vi "VI Interference Konfig.vi"() -> ()   [LabVIEW 2020, in "EPA 1065.lvlib" / "Interference verificaton 1065-375.lvlib"]
uses:
  Interference verificaton 1065-375.lvlib
  Visualisierungs Elemente/Zahlen-Ausgabefeld.ctl
  ResultTable.ctl
  TestKonfig.ctl
  Modus.ctl
  TestSetting.ctl
  Seiten/System Einstellungen V2/Analysatoren.ctl
  Visualisierungs Elemente/String - Ausgabefeld.ctl
  Aktion Test.ctl
  Aktion FGV Interference.ctl
  Linearisierung V2/AktivButton.ctl
  Sprachverwaltung/FGV Aktion Tabelle zerlegen.ctl
  Seiten/FT-IR/FGV FT-IR Gasliste Aktionen.ctl
  Aktion Index uebersetzten.ctl
  Allgemeine VIs/Aktion Test Status.ctl
  Allgemeine VIs/Aktion Wertaenderung Gasliste.ctl
  Messdaten/Aktionen FGV Messdaten.ctl
  Funktionstasten/Zustaende.ctl
  Funktionstasten/Funktionstasten-Aktion.ctl
  <vilib>/Utility/miscctls.llb/LVRowAndColumnTypeDef.ctl
  Seiten/FT-IR/FGV FT-IR Parameter.vi
  Messdaten/Messdaten.lvlib
  Seiten/Grafik/Grafik.lvlib
  Allgemein/allgemeine Sub-VIs.lvlib
  Seiten/FT-IR/FT-IR.lvlib
  Sprachverwaltung/Sprachverwaltung.lvlib
  Funktionstasten/Funktionstasten.lvlib
  Linearisierung V2/Protokoll/Protokoll.lvlib
  Seiten/FT-IR/Span/Spanfaktor.lvlib
  Linearisierung V2/Linearisierung v2.lvlib
  EPA 1065.lvlib
  Seiten/System Einstellungen V2/System Einstellungen V2.lvlib
panel:
  in  "Systemeinstellung":bool caption="Gasliste geändert"
  out "max. Flow Weighted Mean:":T1 caption="ppm"
  out "Konzentration FlowWeightedMean":sgl=120.0 caption="Konzentration:" min=0 format="%#.2f"
  in  "Gasliste vergleichen":bool
  in  "Registerkarte":T2(tab)
  in  "Speichern 2":bool caption="Speichern"
  in  "TestSetting":T3={"Bearbeiter:"="", "Pfad:"=path "D:/IAG_Data/Log", "Textname:"="", "Analysator"=""}
  in  "TestKonfig":T5={"Komponente:"=0, "Modus"=0, "CG Aufschaltzeit:"=120.0, "Interferent 1:"=0, "Interferent 2:"=0, "Interferent 3:"=0, "Gasflaschen Nr.:"="", "Gasflaschen Nr.: 2"="", "Gasflaschen Nr.: 3"="", "Inter 1 aktiv"=FALSE, "Inter 2 aktiv"=FALSE, "Inter 3 aktiv"=FALSE, "Accuracy"="", "Accuracy 2"="", "Accuracy 3"="", "Konzentration 1:"=120.0, "Konzentration 2:"=120.0, "Konzentration 3:"=120.0} {"Komponente:" items=["N2O (300) LP 191C (1of2)", "N2O (1000) LP 191C (2of2)", "N2O autorange (1000)"]; "Konzentration 3:" min=0.0; "Interferent 3:" items=["CO% (1) LP 191C (2of3)", "CO% (10) LP 191C (3of3)", "HNCO (400) 191C", "CO (700) LP 191C (1of3)", "CO autorange (100000)"]; "Konzentration 2:" min=0.0; "Interferent 2:" items=["H2O% (30) LP 191C", "H2Oppm (300000)"]; "Konzentration 1:" min=0.0; "Interferent 1:" items=["CO2 low% (4) LP 191C (2of2)", "CO2% (20) LP 191C (1of2)", "CO2% autorange (20)"]; "Modus" items=["Messen", "CG zu Entnahmestelle"]; "CG Aufschaltzeit:" min=60.0}
  in  "Speichern":bool
  in  "Graph löschen":bool caption="Test Start"
  out "Interferent 3:":T1
  out "Interferent 3: 2":T7 caption="ppm" format="%#.2f"
  out "Interferent 2:":T1
  out "Interferent 2: 2":T7 caption="%" format="%#.2f"
  out "Interferent 1:":T1
  out "Interferent 1: 2":T7 caption="%" format="%#.2f"
  in  "Abbrechen":bool caption="Test Start"
  out "Testdauer":T7
  out "Stabilisierungszeit":T7
  out "Graph":waveform(dbl)[](graph)
  out "Status":string
  in  "Test Start":bool
  out "Komponente 1S:":T1 caption="Komponente:"
  out "Komponente 1:":T7 caption="ppm" format="%#.2f"
  in  "Save to file":bool caption="PDF erstellen"
  out "[ppm]":sgl=1.0 caption="Grenze:" min=0 format="%#.6g"
  out "[ppm]":sgl=120.0 caption="Querempfindlichkeit:" min=0 format="%#.6g"
  out "Konzentration Komponente":sgl=120.0 caption="Konzentration:" min=0 format="%#.2f"
  out "Komponente:":T1 caption="ppm"
  out "LIN Ausgabetabelle":T8
  in  "Daten löschen":bool caption="Test Start"
  in  "Print to PDF":bool caption="PDF erstellen"
  out "Tabelle 3":string[][](table)
  # "N2O Querempfindlichkeitsnachweis 1065.375"
  # "Interference Test"
  # "Interference Verification"
  # "max. Flussgewichteter Mittelwert"
  # "Einstellungen"
  # "General Information"
  # "Report Settings"
  # "Test Einstellungen"
  # "Komponente:"
  # "Interferenten"
  # "sec."
  # "Test"
  # "Ergebnis"
  # "Analyse"
  # "Komponente:"
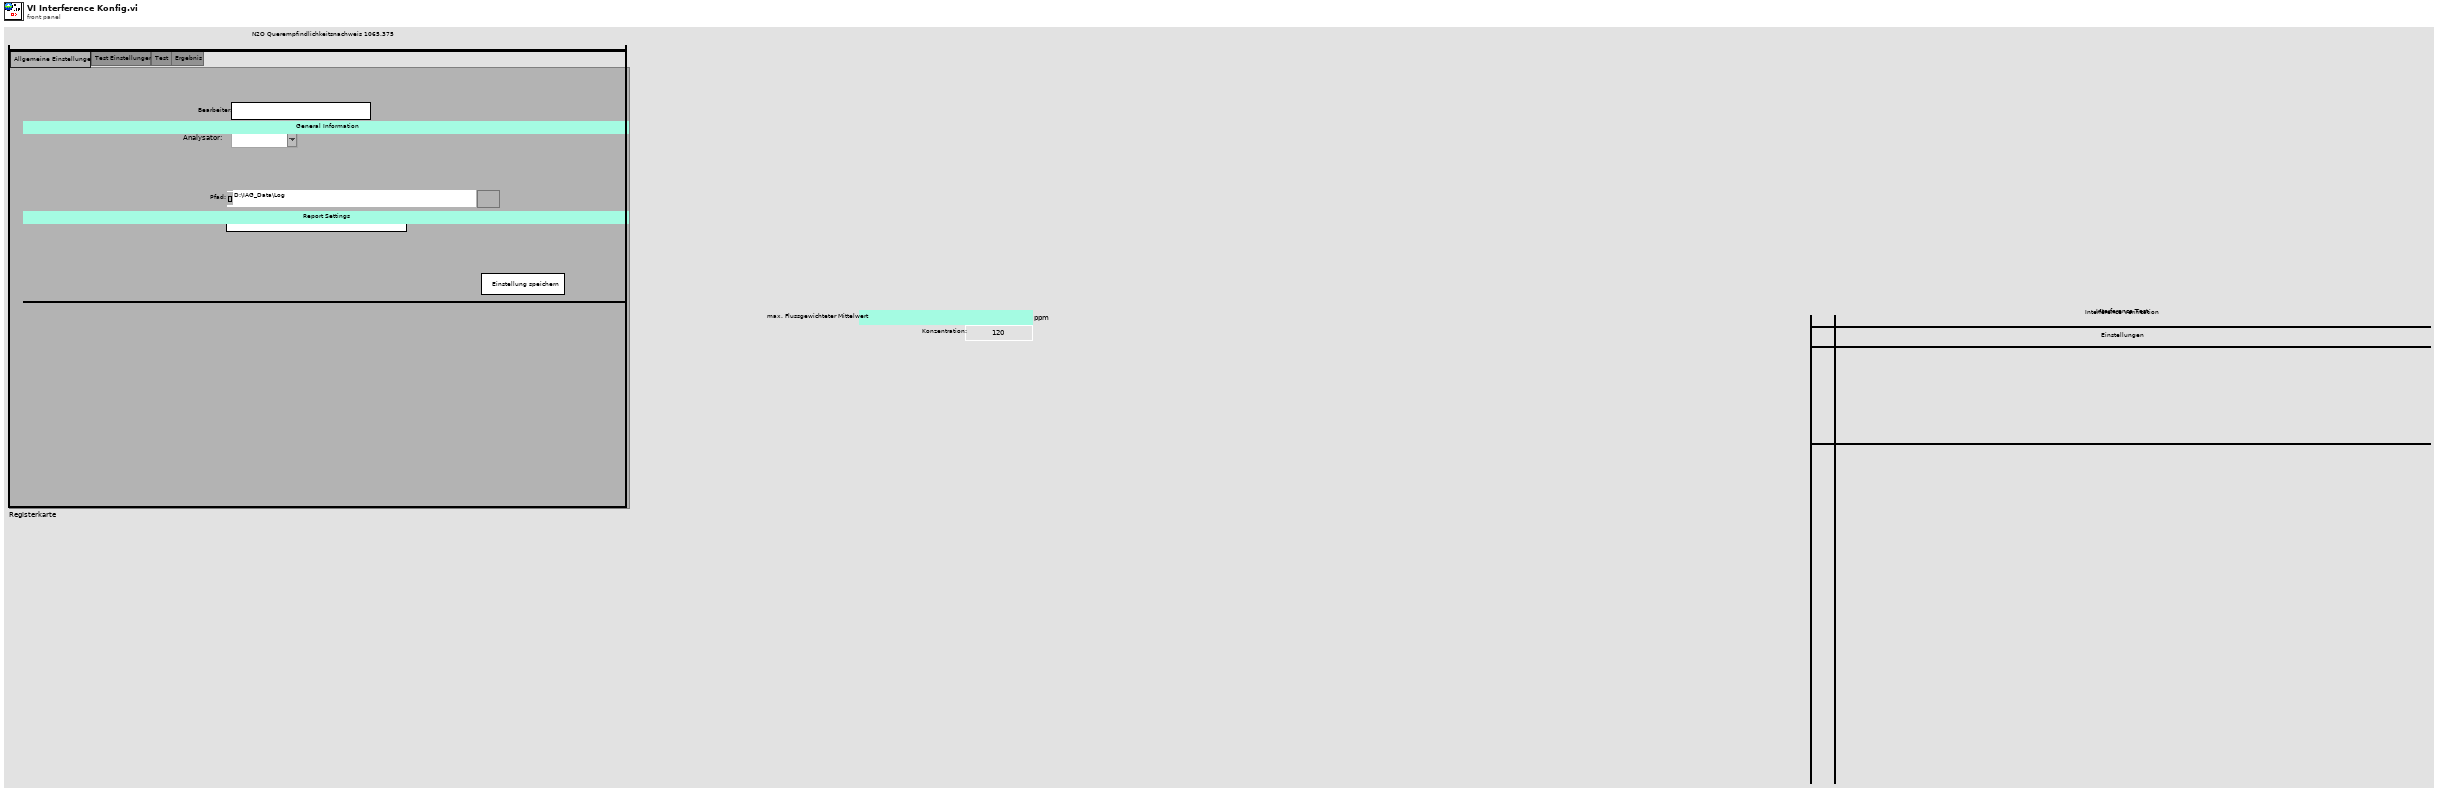
[diagram p1: front panel]
types:
  T1 = typedef "String - Ausgabefeld.ctl" = string
  T2 = enum32{"General Settings", "Test Settings", "Test", "Result"}
  T3 = typedef "EPA 1065.lvlib/Interference verificaton 1065-375.lvlib/TestSetting.ctl" = cluster{"Bearbeiter:":string, "Pfad:":path, "Textname:":string, "Analysator":T4}
  T4 = typedef "System Einstellungen V2.lvlib/Analysatoren.ctl" = string
  T5 = typedef "EPA 1065.lvlib/Interference verificaton 1065-375.lvlib/TestKonfig.ctl" = cluster{"Komponente:":u16, "Modus":T6, "CG Aufschaltzeit:":dbl, "Interferent 1:":u16, "Interferent 2:":u16, "Interferent 3:":u16, "Gasflaschen Nr.:":string, "Gasflaschen Nr.: 2":string, "Gasflaschen Nr.: 3":string, "Inter 1 aktiv":bool, "Inter 2 aktiv":bool, "Inter 3 aktiv":bool, "Accuracy":string, "Accuracy 2":string, "Accuracy 3":string, "Konzentration 1:":dbl, "Konzentration 2:":dbl, "Konzentration 3:":dbl}
  T6 = typedef "EPA 1065.lvlib/Interference verificaton 1065-375.lvlib/Modus.ctl" = u16
  T7 = typedef "Zahlen-Ausgabefeld.ctl" = sgl
  T8 = typedef "EPA 1065.lvlib/Interference verificaton 1065-375.lvlib/ResultTable.ctl" = string[][]
  T9 = typedef "EPA 1065.lvlib/Interference verificaton 1065-375.lvlib/Aktion Test.ctl" = enum16{"Lesen", "ini", "ini - Konz", "Konzentration erreicht", "ini-warten", "ini-Warten-Stabil", "Warten-Stabil", "ini-warten-aufzeichnen", "Warten-Aufzeichnen", "aufzeichnen", "ini-wet", "ini - konz - wet", "Konzentration erreicht - wet", "ini - warten - wet", "warten - wet", "warten - aufzeichnen - wet", "Auswerten", "aufzeichnen - wet"}
  T10 = typedef "Sprachverwaltung.lvlib/FGV Aktion Tabelle zerlegen.ctl" = enum16{"laden", "vereinzeln", "speichern"}
  T11 = typedef "Linearisierung v2.lvlib/AktivButton.ctl" = bool
  T12 = typedef "EPA 1065.lvlib/Interference verificaton 1065-375.lvlib/Aktion FGV Interference.ctl" = enum16{"Lesen", "TestKonfig", "TestSetting", "Einheiten", "Ergebnis", "Laden", "Tabelle", "Speichern", "löschen"}
  T13 = enum8{"Enabled", "Disabled", "Disabled and Grayed Out"}
  T14 = typedef "EPA 1065.lvlib/Interference verificaton 1065-375.lvlib/Aktion Index uebersetzten.ctl" = enum16{"lesen", "schreiben", "auswerten"}
  T15 = typedef "FT-IR.lvlib/FGV FT-IR Gasliste Aktionen.ctl" = enum16{"lesen", "Gasliste FT-IR", "Gasliste ausgelesen", "laden", "speichern", "löschen"}
  T16 = typedef "EPA 1065.lvlib/Interference verificaton 1065-375.lvlib/Komponenten.ctl" = cluster{"Komponente":T1, "Komponente Index":i32, "Komponente 2":T1, "Komponente Index 2":i32, "Komponente 3":T1, "Komponente Index 3":i32, "Interferent 1":T1, "Interferent Index":i32, "Interferent 2":T1, "Interferent 2 Index":i32, "Interferent 3":T1, "Interferent 3 Index":i32, "Interferent 4":T1, "Interferent 4 Index":i32}
  T17 = typedef "EPA 1065.lvlib/Aktion Wertaenderung Gasliste.ctl" = enum16{"Init", "lesen", "Gasliste geändert", "ARN inaktiv", "LEAK inaktiv", "Interference 366 inaktiv", "T90 inaktiv", "Interference 375 inaktiv", "Chiller inaktiv", "FID O2 inaktiv", "FID Opti inaktiv", "Drift inaktiv", "Pre Test inaktiv", "LinV2 inaktiv", "HovaCAL Interference inaktiv"}
  T18 = typedef "EPA 1065.lvlib/Aktion Test Status.ctl" = enum16{"init", "lesen", "prüfen", "Interference 366", "Interference 375", "Chiller läuft", "Drift läuft", "Pre Test läuft", "FID Optimization läuft", "FID Interference läuft", "HovaCAL Interference", "LinV2"}
  T19 = typedef "Messdaten.lvlib/Aktionen FGV Messdaten.ctl" = enum16{"lesen", "schreiben", "löschen", "Mittelwerte", "Komponente"}
  T20 = typedef "Funktionstasten.lvlib/Funktionstasten-Aktion.ctl" = enum16{"Initialisieren", "Zustand setzen", "Taste gedrückt", "Fehler speichern", "Lesen", "Manuell", "Remote", "Bitparallel", "Samplepoint", "Zeit Prüfen", "reset Umschalten"}
  T21 = typedef "Funktionstasten.lvlib/Zustaende.ctl" = enum16{"Standby", "Pause", "Eco", "Messen", "Kalibrieren", "Spülen Filter", "Spülen Leitung", "Umgebungsluft", "0-Gas", "Cal-Gas", "CG zu PNS", "-------------", "Init 1", "Init 2", "Init 3", "Init 4", "Messen vorbereiten", "Messen durchführen", "Exit"}
  T22 = enum16{"open", "replace", "create", "open or create", "replace or create", "replace or create with confirmation"}
  T23 = typedef "LVRowAndColumnTypeDef.ctl" = cluster{"Row":i32, "Column":i32}
  T24 = typedef "EPA 1065.lvlib/Aktive Tests Cluster.ctl" = cluster{"ANR läuft":bool, "T90 läuft":bool, "Leak läuft":bool, "Interference 366 läuft":bool, "Interference 375 läuft":bool, "Chiller läuft":bool, "FID Interference läuft":bool, "FID optimization läuft":bool, "Drift läuft":bool, "Pre-test läuft":bool, "HovaCAL Interference läuft":bool, "LinV2 läuft":bool}
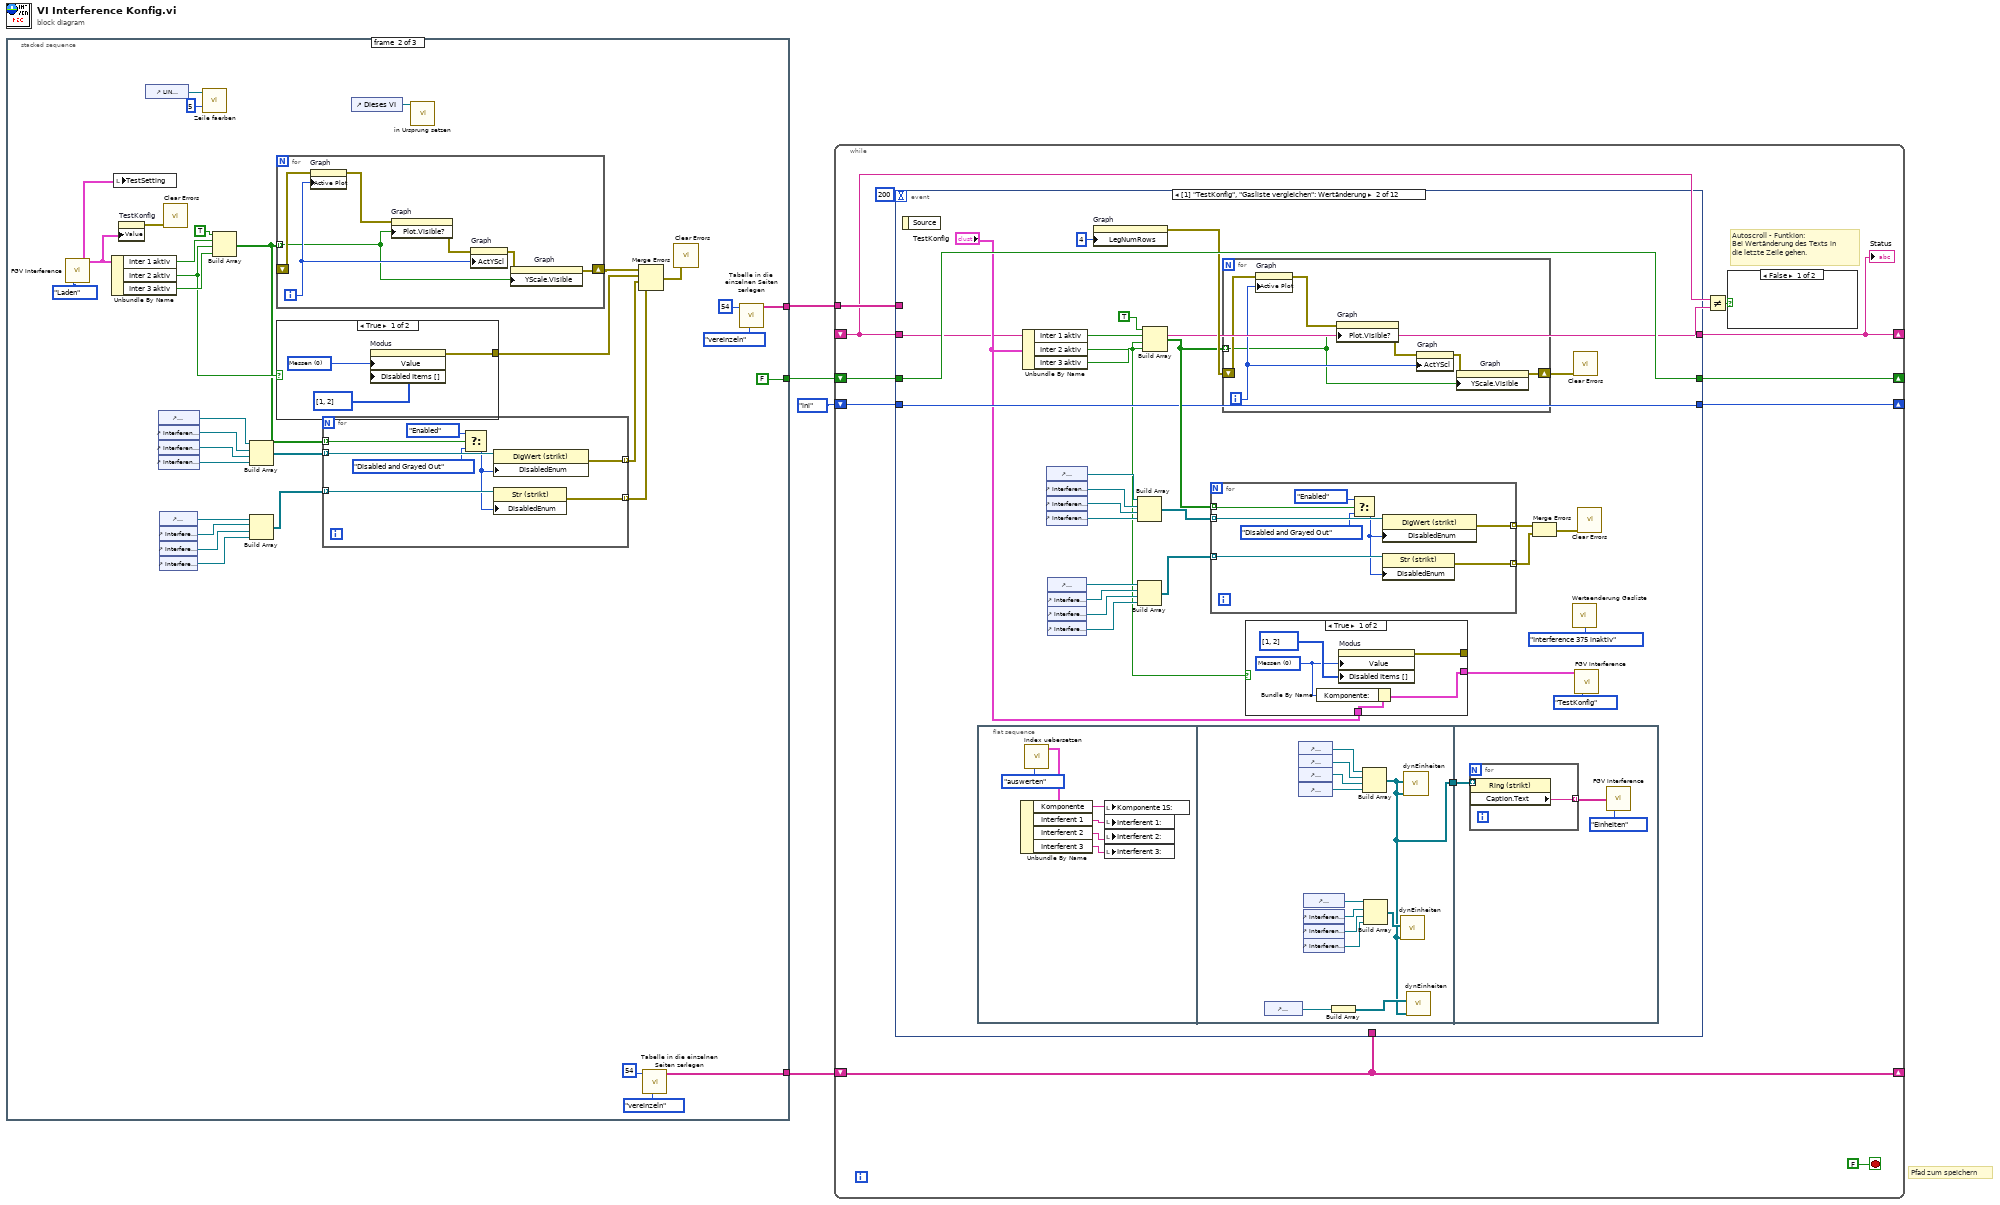
[diagram p0: block diagram]
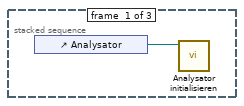
[diagram p2: hidden frame]
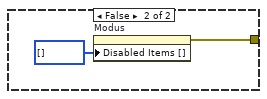
[diagram p3: hidden frame]
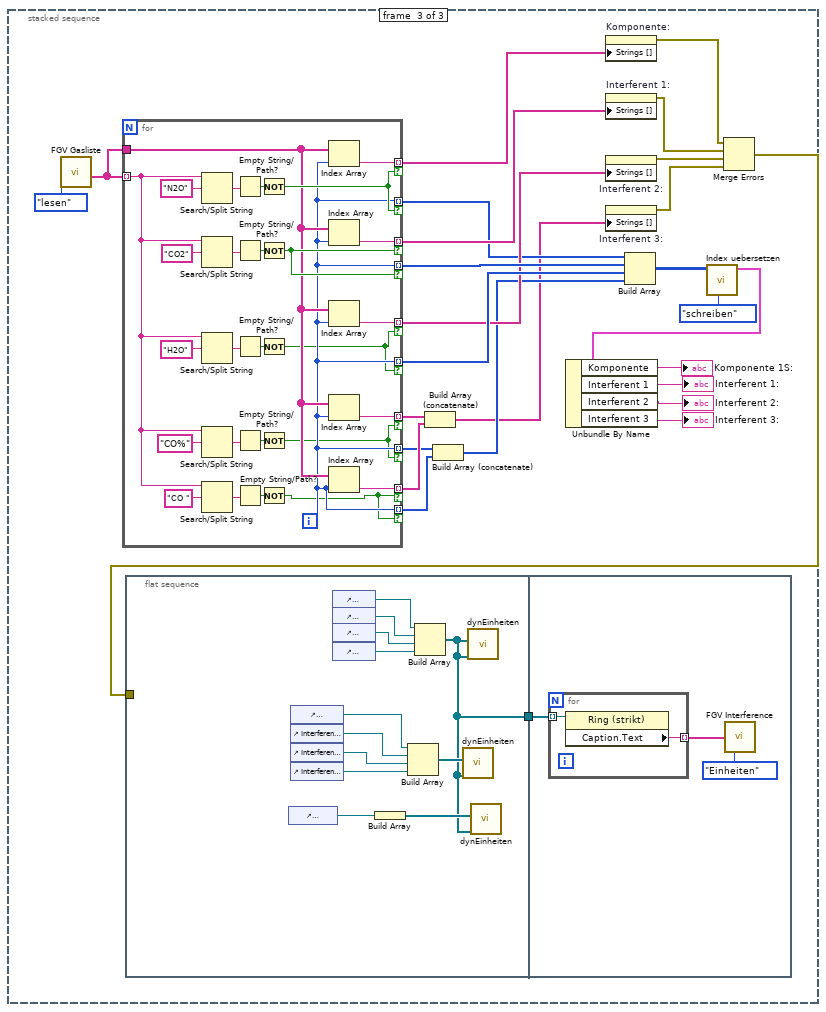
[diagram p4: hidden frame]
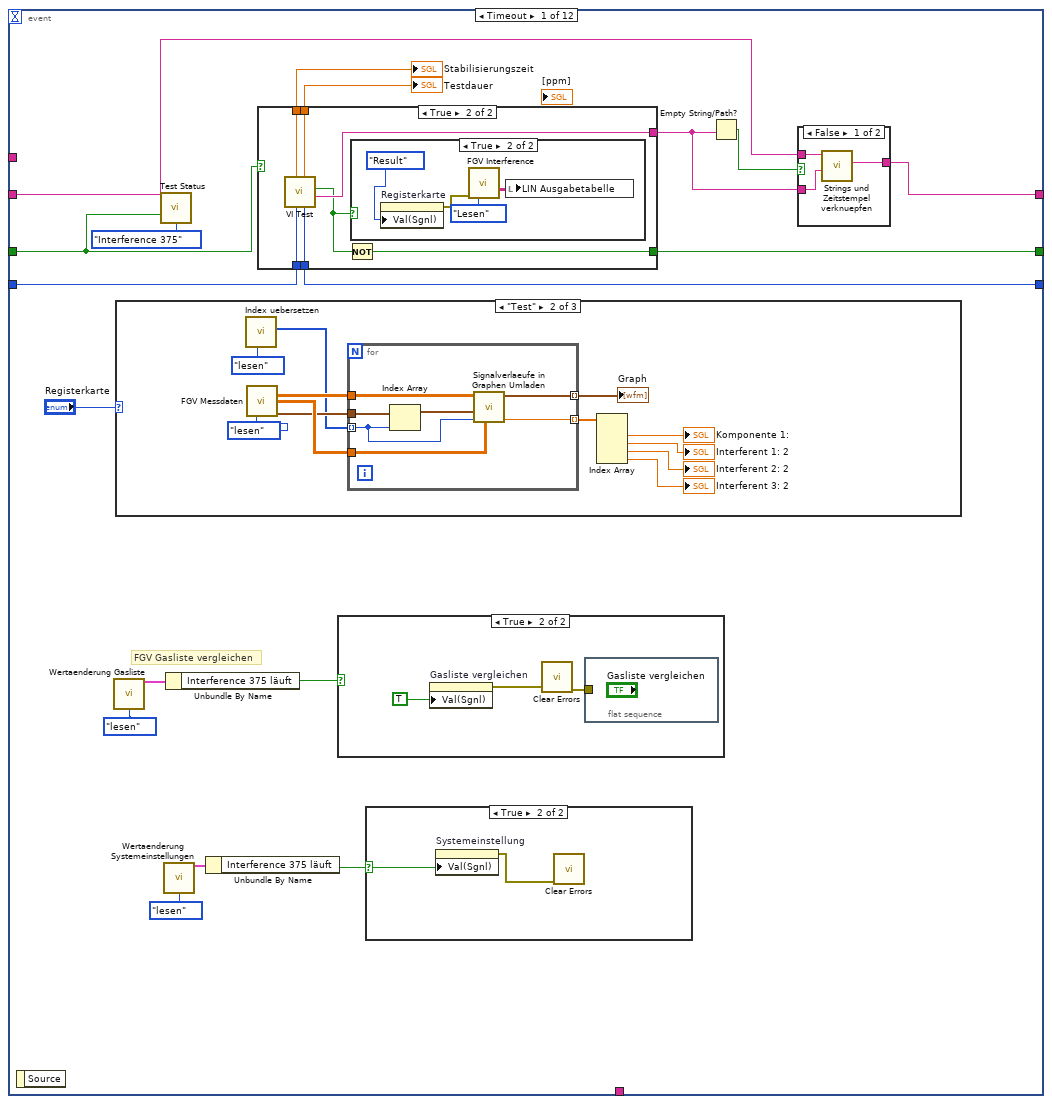
[diagram p5: hidden frame]
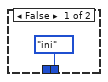
[diagram p10: hidden frame]
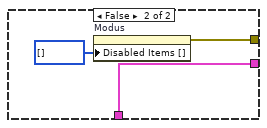
[diagram p13: hidden frame]
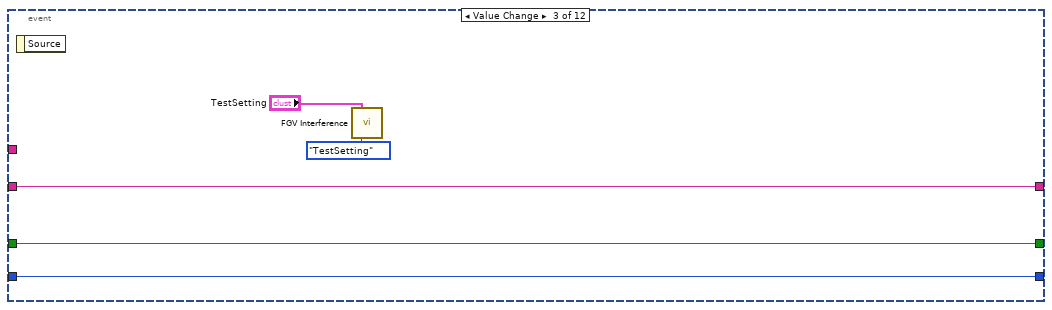
[diagram p14: hidden frame]
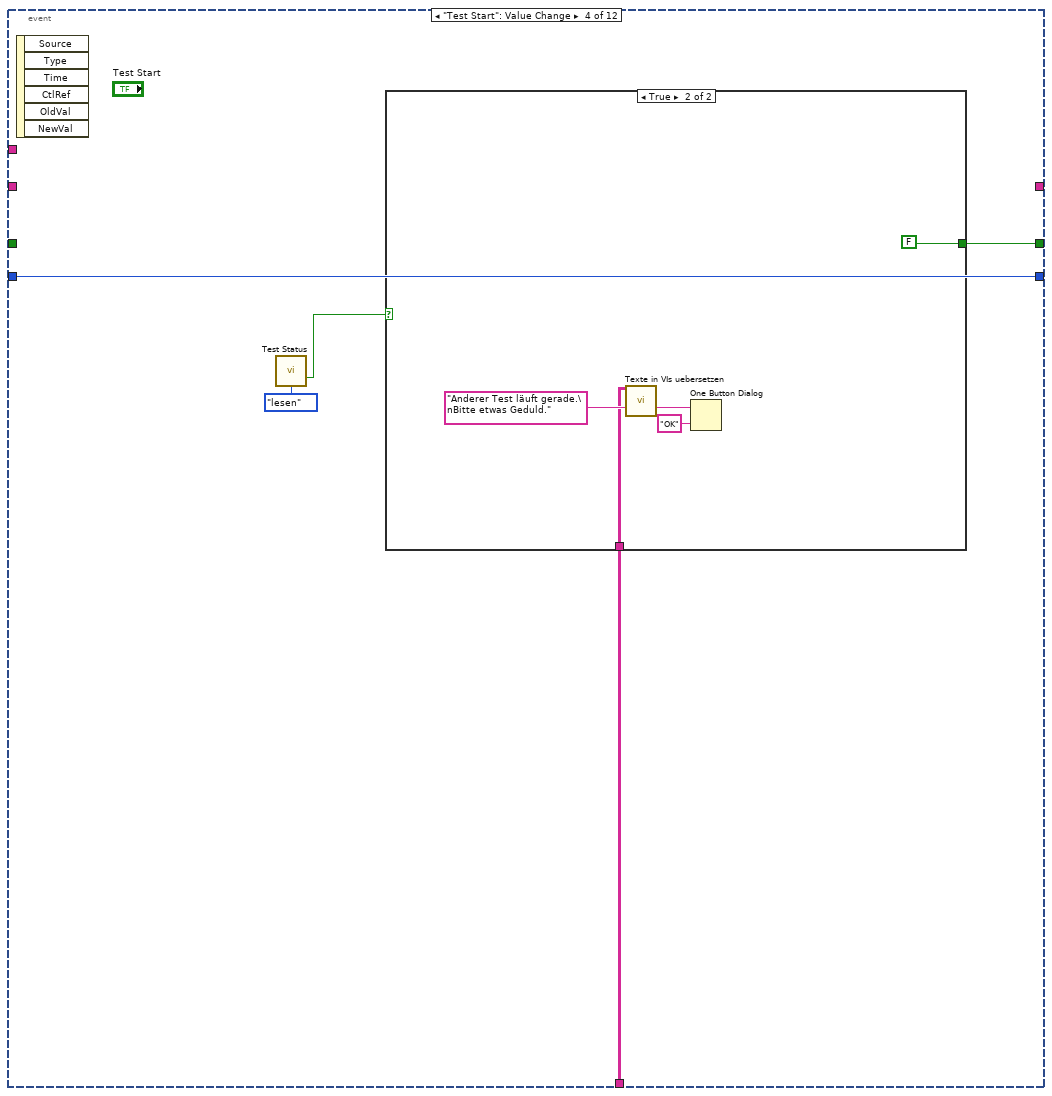
[diagram p15: hidden frame]
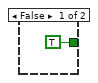
[diagram p16: hidden frame]
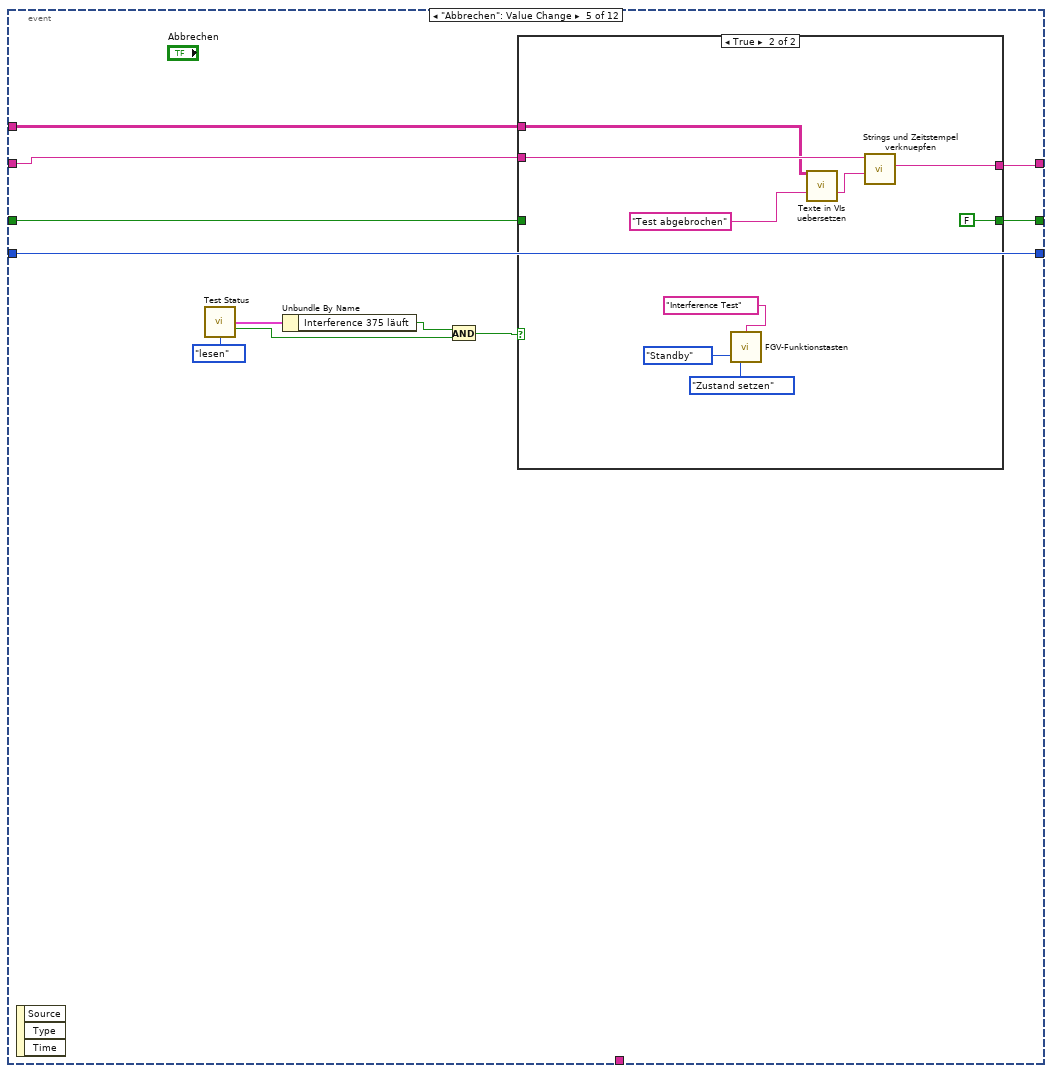
[diagram p17: hidden frame]
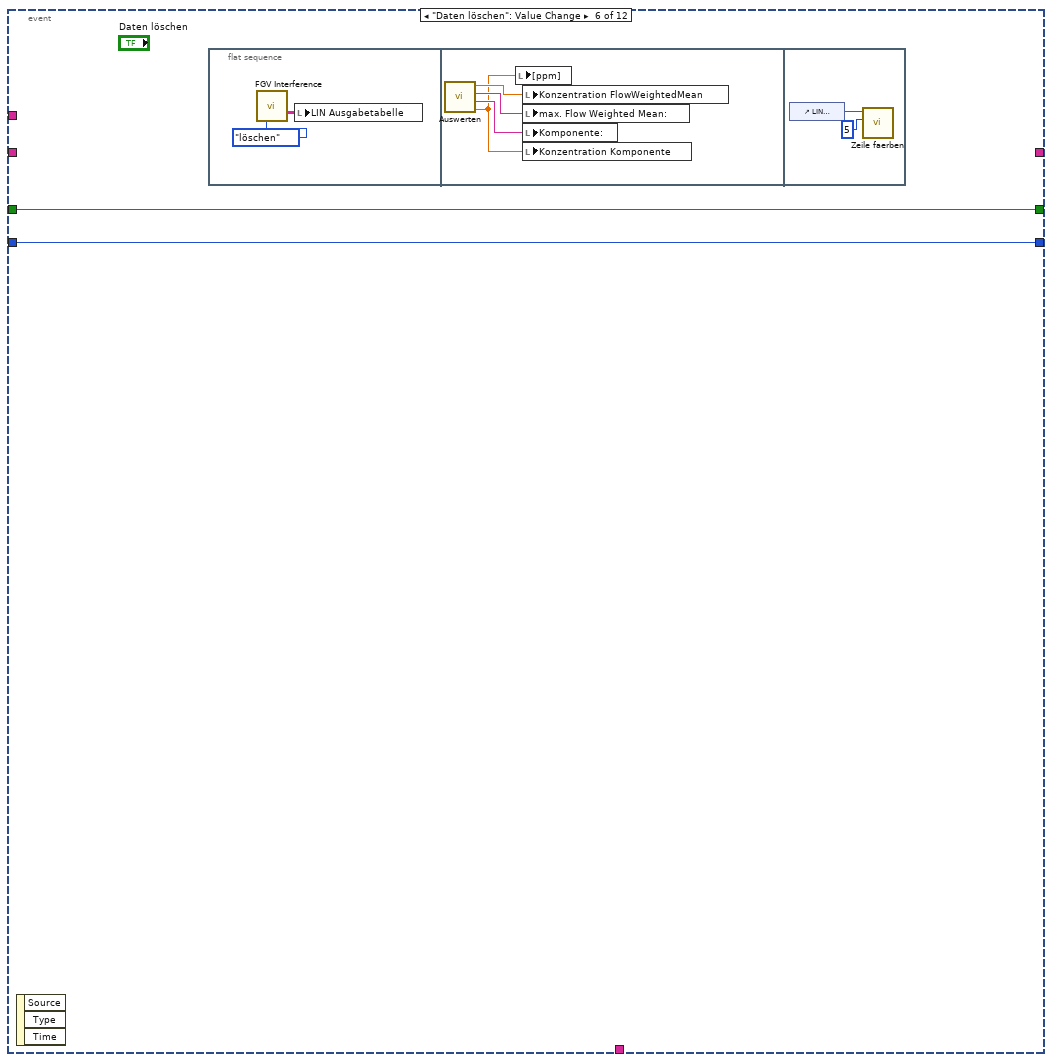
[diagram p19: hidden frame]
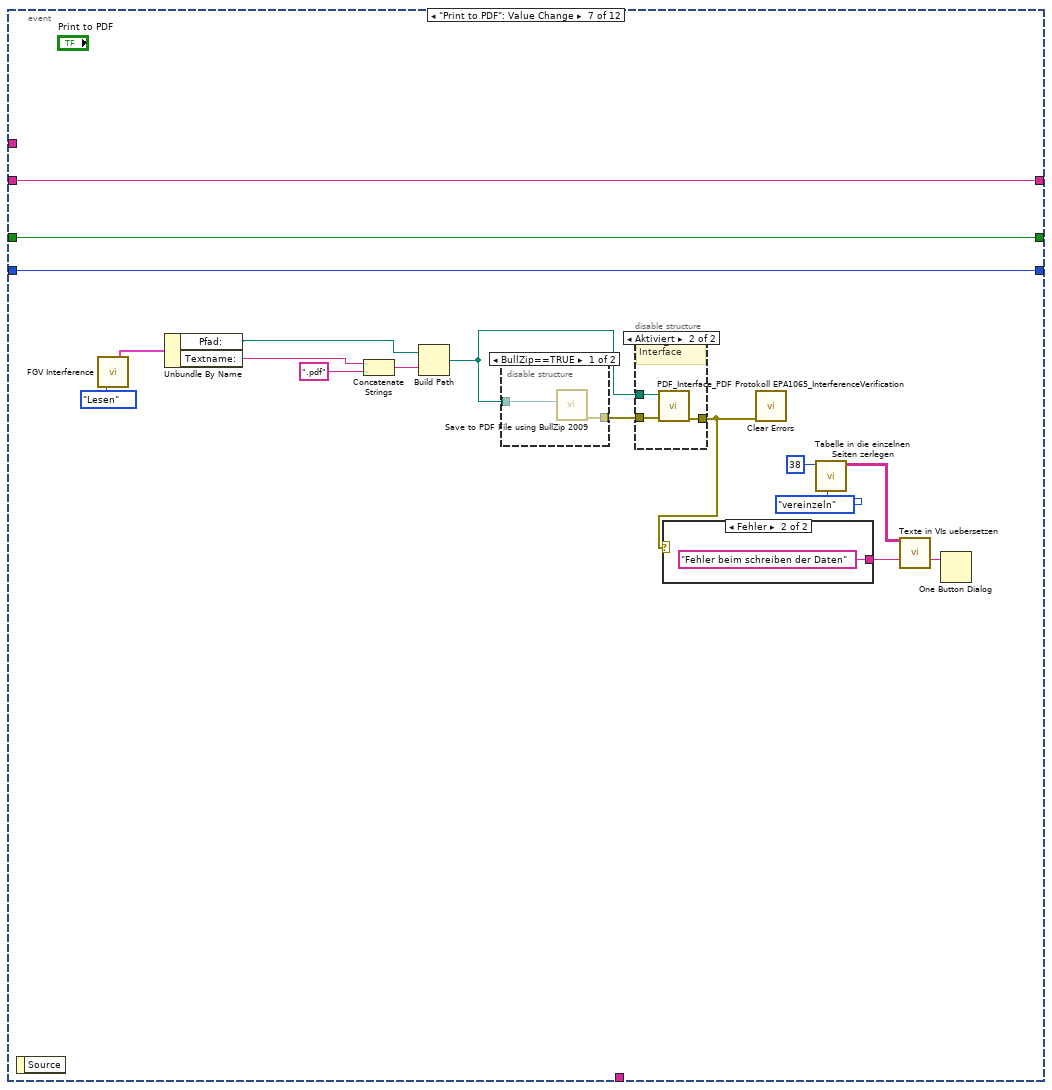
[diagram p20: hidden frame]
diagram:
  # "Pfad zum speichern"
  n1 = stacked-sequence {
    tunnel: [_ w37 _] -> w4
    tunnel: [_ FALSE _] -> w3
    tunnel: [_ w19 _] -> w1
    frame #0 {
      n2 = control-ref of="Analysator"() -> (w5:refnum<vi>)
      n3 = call "Analysator initialisieren.vi"("Referenz Analysator"=w5) -> ()  [unwired: 9 in, 2 out]
    }
    frame #1 {
      n4 = call "FGV Interference.vi"("Aktion FGV Interference"=Aktion_FGV_Interference."Laden") -> ("TestSetting"=w30:T3, "TestKonfig 2"=w34:T5)  [unwired: 9 in, 4 out]
      n5 = Unbundle By Name(w34) -> ("Inter 1 aktiv"=w29:bool, "Inter 2 aktiv"=w25:bool, "Inter 3 aktiv"=w28:bool)
      n6 = local write "TestSetting"(w30) -> ()
      n7 = property on="TestKonfig" class="Cluster (strikt)"("Value"=w34) -> (error out=w33:errorcluster)  [unwired: 2 in, 1 out]
      n8 = control-ref of="LIN Ausgabetabelle"() -> (w31:refnum<vi>)
      n9 = control-ref of="Komponente 1:"() -> (w12:refnum<vi>)
      n10 = control-ref of="Interferent 1: 2"() -> (w11:refnum<vi>)
      n11 = control-ref of="Interferent 2: 2"() -> (w10:refnum<vi>)
      n12 = control-ref of="Interferent 3: 2"() -> (w9:refnum<vi>)
      n13 = control-ref of="Komponente 1S:"() -> (w13:refnum<vi>)
      n14 = control-ref of="Interferent 1:"() -> (w14:refnum<vi>)
      n15 = control-ref of="Interferent 2:"() -> (w15:refnum<vi>)
      n16 = control-ref of="Interferent 3:"() -> (w16:refnum<vi>)
      n17 = call <vilib>:"Clear Errors.vi"("error in (no error)"=w33) -> ()  [unwired: 5 in, 2 out]
      n18 = call "Zeile faerben.vi"("Anzahl"=5, "Table (Eingang)"=w31) -> ()  [unwired: 9 in, 1 out]
      n19 = Build Array(T11 TRUE ("Element"), w29, w25, w28) -> (w8:T11[])
      n20 = Build Array(w12, w11, w10, w9) -> (w17:refnum<vi>[])
      n21 = Build Array(w13, w14, w15, w16) -> (w18:refnum<vi>[])
      n22 = for {
        shift-right: [w56] -> w24
        shift-left: _ -> [w55]
        tunnel: w8 -> [w53] mode=indexing
        i -> [w54]
        n23 = property on="Graph" class="SVDiagr (strikt)"(error in=w55, "Active Plot"=w54) -> (error out=w57:errorcluster)  [unwired: 1 in, 1 out]
        n24 = property on="Graph" class="SVDiagr (strikt)"(error in=w57, "Plot.Visible?"=w53) -> (error out=w58:errorcluster)  [unwired: 1 in, 1 out]
        n25 = property on="Graph" class="SVDiagr (strikt)"(error in=w58, "ActYScl"=w54) -> (error out=w59:errorcluster)  [unwired: 1 in, 1 out]
        n26 = property on="Graph" class="SVDiagr (strikt)"(error in=w59, "YScale.Visible"=w53) -> (error out=w56:errorcluster)  [unwired: 1 in, 1 out]
      }
      n27 = case shown="True" w25 {
        tunnel: [w48 w51] -> w22
        frame True {
          w50 = T6 0 items=["Messen", "CG zu PNS", "CG zu Entnahmestelle"] ("Wert")
          n28 = property on="Modus" class="Ring (strikt)"("Value"=w50, "Disabled Items []"=i32[] [1, 2] ("Deaktivierte Objekte []")) -> (error out=w48:errorcluster)  [unwired: 2 in, 1 out]
        }
        frame False {
          n29 = property on="Modus" class="Ring (strikt)"("Disabled Items []"=i32[] [] ("Deaktivierte Objekte []")) -> (error out=w51:errorcluster)  [unwired: 2 in, 1 out]
        }
      }
      n30 = for {
        tunnel: w8 -> [w40] mode=indexing
        tunnel: w17 -> [w47] mode=indexing
        tunnel: w18 -> [w46] mode=indexing
        tunnel: [w45] -> w7 mode=indexing
        tunnel: [w44] -> w6 mode=indexing
        n31 = Select(t=T13."Enabled" ("Deaktiviert"), s=w40, f=T13."Disabled and Grayed Out" ("Deaktiviert")) -> (s? t:f=w41:T13)
        n32 = property class="DigWert (strikt)"(reference=w47, "DisabledEnum"=w41) -> (error out=w45:errorcluster)  [unwired: 1 in, 1 out]
        n33 = property class="Str (strikt)"(reference=w46, "DisabledEnum"=w41) -> (error out=w44:errorcluster)  [unwired: 1 in, 1 out]
      }
      n34 = control-ref of="Dieses VI"() -> (w39:refnum<vi>)
      n35 = call "in Ursprung setzen.vi"("VI Referenz"=w39) -> ()  [unwired: 10 in, 1 out]
      n36 = Merge Errors(w24, w22, w7, w6) -> (w23:errorcluster)
      n37 = call "Tabelle in die einzelnen Seiten zerlegen.vi"("Aktion"=FGV_Aktion_Tabelle_zerlegen."vereinzeln", "Index (Seite)"=54) -> ("Sprachliste"=w19:string[][])  [unwired: 7 in, 2 out]
      n38 = call <vilib>:"Clear Errors.vi"("error in (no error)"=w23) -> ()  [unwired: 5 in, 2 out]
      n39 = call "Tabelle in die einzelnen Seiten zerlegen.vi"("Aktion"=FGV_Aktion_Tabelle_zerlegen."vereinzeln", "Index (Seite)"=54) -> ("Sprachliste"=w37:string[][])  [unwired: 7 in, 2 out]
    }
    frame #2 {
      n40 = call "FGV Gasliste.vi"("Aktionen"=FGV_FT-IR_Gasliste_Aktionen."lesen") -> ("Aktuelle Gasliste gesamt"=w83:T1[])  [unwired: 8 in, 2 out]
      n41 = for {
        tunnel: w83 -> [w110] mode=indexing
        tunnel: w83 -> [w109]
        tunnel: [w128] -> w69 mode=indexing if=w127
        tunnel: [w107] -> w66 mode=indexing if=w127
        tunnel: [w125] -> w68 mode=indexing if=w126
        tunnel: [w107] -> w73 mode=indexing if=w126
        tunnel: [w118] -> w67 mode=indexing if=w105
        tunnel: [w107] -> w84 mode=indexing if=w105
        tunnel: [w117] -> w65 mode=indexing if=w106
        tunnel: [w107] -> w63 mode=indexing if=w106
        tunnel: [w108] -> w64 mode=indexing if=w104
        tunnel: [w107] -> w62 mode=indexing if=w104
        i -> [w107]
        n42 = Search/Split String(string=w110, search string/char (-)="N2O" ("Such-String/-Zeichen (-)")) -> (match + rest of string=w130:T1)  [unwired: 1 in, 2 out]
        n43 = Search/Split String(string=w110, search string/char (-)="CO2" ("Such-String/-Zeichen (-)")) -> (match + rest of string=w123:T1)  [unwired: 1 in, 2 out]
        n44 = Search/Split String(string=w110, search string/char (-)="H2O" ("Such-String/-Zeichen (-)")) -> (match + rest of string=w120:T1)  [unwired: 1 in, 2 out]
        n45 = Search/Split String(string=w110, search string/char (-)="CO%" ("Such-String/-Zeichen (-)")) -> (match + rest of string=w115:T1)  [unwired: 1 in, 2 out]
        n46 = Search/Split String(string=w110, search string/char (-)="CO " ("Such-String/-Zeichen (-)")) -> (match + rest of string=w112:T1)  [unwired: 1 in, 2 out]
        n47 = Empty String/Path?(string/path=w130) -> (empty?=w131:bool)
        n48 = Empty String/Path?(string/path=w123) -> (empty?=w122:bool)
        n49 = Empty String/Path?(string/path=w120) -> (empty?=w121:bool)
        n50 = Empty String/Path?(string/path=w115) -> (empty?=w114:bool)
        n51 = Empty String/Path?(string/path=w112) -> (empty?=w113:bool)
        n52 = Not(x=w131) -> (.not. x?=w127:bool)
        n53 = Not(x=w122) -> (.not. x?=w126:bool)
        n54 = Not(x=w121) -> (.not. x?=w105:bool)
        n55 = Not(x=w114) -> (.not. x?=w106:bool)
        n56 = Not(x=w113) -> (.not. x?=w104:bool)
        n57 = Index Array(array=w109, index=w107) -> (element=w128:T1)
        n58 = Index Array(array=w109, index=w107) -> (element=w125:T1)
        n59 = Index Array(array=w109, index=w107) -> (element=w118:T1)
        n60 = Index Array(array=w109, index=w107) -> (element=w117:T1)
        n61 = Index Array(array=w109, index=w107) -> (element=w108:T1)
      }
      n62 = flat-sequence {
        tunnel: w82 -> [_]
        tunnel: [w91] -> w86
        tunnel: w86 -> [w101]
        frame #0 {
          n63 = control-ref of="Komponente:"() -> (w92:refnum<vi>)
          n64 = control-ref of="Komponente 1:"() -> (w88:refnum<vi>)
          n65 = control-ref of="Interferent 1: 2"() -> (w87:refnum<vi>)
          n66 = control-ref of="Interferent 2: 2"() -> (w95:refnum<vi>)
          n67 = control-ref of="Interferent 3: 2"() -> (w96:refnum<vi>)
          n68 = control-ref of="Komponente:"() -> (w90:refnum<vi>)
          n69 = control-ref of="Interferent 1:"() -> (w89:refnum<vi>)
          n70 = control-ref of="Interferent 2:"() -> (w98:refnum<vi>)
          n71 = control-ref of="Interferent 3:"() -> (w97:refnum<vi>)
          n72 = Build Array(w92) -> (w93:refnum<vi>[])
          n73 = Build Array(w88, w87, w95, w96) -> (w94:refnum<vi>[])
          n74 = Build Array(w90, w89, w98, w97) -> (w91:refnum<vi>[])
          n75 = call "dynEinheiten.vi"("Komponenten Ref."=w91, "Sollwert Ref."=w94) -> ()  [unwired: 10 in]
          n76 = call "dynEinheiten.vi"("Komponenten Ref."=w91, "Sollwert Ref."=w91) -> ()  [unwired: 10 in]
          n77 = call "dynEinheiten.vi"("Komponenten Ref."=w91, "Sollwert Ref."=w93) -> ()  [unwired: 10 in]
        }
        frame #1 {
          n78 = for {
            tunnel: w101 -> [w103] mode=indexing
            tunnel: [w102] -> w99 mode=indexing
            n79 = property class="Ring (strikt)"(reference=w103) -> ("Caption.Text"=w102:string)  [unwired: 1 in, 2 out]
          }
          n80 = call "FGV Interference.vi"("Êinheiten"=w99, "Aktion FGV Interference"=Aktion_FGV_Interference."Einheiten") -> ()  [unwired: 8 in, 6 out]
        }
      }
      n81 = Build Array (concatenate)(w65, w64) -> (w60:T1[])
      n82 = Build Array (concatenate)(w63, w62) -> (w61:i32[])
      n83 = property on="Komponente:" class="Ring (strikt)"("Strings []"=w69) -> (error out=w72:errorcluster)  [unwired: 2 in, 1 out]
      n84 = property on="Interferent 1:" class="Ring (strikt)"("Strings []"=w68) -> (error out=w71:errorcluster)  [unwired: 2 in, 1 out]
      n85 = property on="Interferent 2:" class="Ring (strikt)"("Strings []"=w67) -> (error out=w80:errorcluster)  [unwired: 2 in, 1 out]
      n86 = property on="Interferent 3:" class="Ring (strikt)"("Strings []"=w60) -> (error out=w81:errorcluster)  [unwired: 2 in, 1 out]
      n87 = Build Array(w66, w73, w84, w61) -> (w85:i32[][])
      n88 = call "Index uebersetzen.vi"("Aktion"=Aktion_Index_uebersetzten."schreiben", "Array"=w85) -> ("Komponenten"=w77:T16)  [unwired: 8 in, 1 out]
      n89 = Unbundle By Name(w77) -> ("Komponente"=→"Komponente 1S:":T1, "Interferent 1"=→"Interferent 1:":T1, "Interferent 2"=→"Interferent 2:":T1, "Interferent 3"=→"Interferent 3:":T1)
      n90 = Merge Errors(w72, w71, w80, w81) -> (w82:errorcluster)
    }
  }
  n91 = while {
    shift-right: [w139] -> _
    shift-left: w3 -> [w140]
    shift-right: [w135] -> _
    shift-left: _ -> [w137]
    tunnel: w4 -> [w138]
    shift-right: [w134] -> _
    shift-left: Aktion_Test."ini" ("Aktion") -> [w133]
    shift-right: [w132] -> _
    shift-left: w1 -> [w132]
    stop <- FALSE stop-if-true
    # "Autoscroll - Funtkion:\nBei Wertänderung des Texts in \ndie letzte Zeile gehen."
    n92 = event shown="[1] \"TestKonfig\", \"Gasliste vergleichen\": Wertänderung" {
      selector: _ -> [_ _ _ _ _ _ _ _ _ _ _ _]
      dyn-events: _ -> [_ _ _ _ _ _ _ _ _ _ _ _]
      timeout: 200 -> [_ _ _ _ _ _ _ _ _ _ _ _]
      tunnel: [w158 w201 w276 _ w302 _ w338 w350 w356 w380 w384 w390] -> w135
      tunnel: w137 -> [w157 w201 w276 _ w301 _ w338 w350 w356 w380 w384 w390]
      tunnel: w140 -> [w149 w229 w277 _ w292 w315 w337 w352 w358 w382 w386 w405]
      tunnel: [w154 w229 w277 w285 w299 w315 w337 w352 w358 w382 w386 w405] -> w139
      tunnel: w138 -> [_ _ _ _ w298 _ _ _ _ _ _ w392]
      tunnel: [w156 w207 w278 w284 w300 w314 w336 w351 w357 w381 w385 w406] -> w134
      tunnel: w133 -> [w155 w207 w278 w284 w300 w314 w336 w351 w357 w381 w385 w406]
      tunnel: w132 -> [_ _ _ w281 _ _ _ _ _ _ _ _]
      event Timeout {
        # "FGV Gasliste vergleichen"
        n93 = event-data() -> ()  [unwired: 1 in, 1 out]
        n94 = call "Wertaenderung Gasliste.vi"("Aktion"=Aktion_Wertaenderung_Gasliste."lesen") -> ("Tests"=w147:T24)  [unwired: 13 in, 1 out]
        n95 = case shown="\"Test\"" "Registerkarte" {
          frame "General Settings", Default {
          }
          frame "Test" {
            n96 = call "Index uebersetzen.vi"("Aktion"=Aktion_Index_uebersetzten."lesen") -> ("Komponenten"=w172:i32[])  [unwired: 9 in, 1 out]
            n97 = call "FGV Messdaten.vi"("Aktionen"=Aktionen_FGV_Messdaten."lesen") -> ("Messdaten"=w173:sgl[][], "Mittelwertdaten"=w175:sgl[][], "Zeitstempeln"=w174:timestamp[])  [unwired: 6 in, 6 out]
            n98 = for {
              tunnel: w175 -> [w184]
              tunnel: w174 -> [w183]
              tunnel: w173 -> [w181]
              tunnel: w172 -> [w180] mode=indexing
              tunnel: [w179] -> w171 mode=indexing
              tunnel: [w178] -> w170 mode=indexing
              n99 = Index Array(array=w183, index=w180) -> (element=w182:timestamp)
              n100 = call "Signalverlaeufe in Graphen Umladen.vi"("Mittelwertdaten"=w184, "Gas-Auswahl"=w180, "t0"=w182, "Werte"=w181) -> ("Konzentration"=w178:sgl, "Waveform"=w179:waveform(dbl))  [unwired: 3 in, 3 out]
            }
            "Graph" <- w171
            n101 = Index Array(array=w170) -> (element #1=→"Komponente 1:":sgl, element #2=→"Interferent 1: 2":sgl, element #3=→"Interferent 2: 2":sgl, element #4=→"Interferent 3: 2":sgl)  [unwired: 4 in]
          }
          frame "Result" {
          }
        }
        n102 = call "Test Status.vi"("Interference 375 läuft"=w149, "Aktion"=Aktion_Test_Status."Interference 375") -> ()  [unwired: 10 in, 4 out]
        n103 = call "Wertaenderung Systemeinstellungen.vi"("Aktion"=Aktion_Wertaenderung_Gasliste."lesen") -> ("Tests"=w144:T24)  [unwired: 13 in, 1 out]
        n104 = Unbundle By Name(w147) -> ("Interference 375 läuft"=w146:bool)
        n105 = Unbundle By Name(w144) -> ("Interference 375 läuft"=w143:bool)
        n106 = case shown="True" w149 {
          tunnel: [_ w192] -> w159
          tunnel: [Aktion_Test."ini" ("Aktion") w191] -> w156
          tunnel: w155 -> [_ w190]
          tunnel: [_ w189] -> w154
          tunnel: [_ w188] -> w153
          tunnel: [_ w187] -> w152
          frame False {
          }
          frame True {
            n107 = call "VI Test.vi"("Aktion"=w190) -> ("Status Test"=w192:string, "Fertig"=w186:bool, "Aktion"=w191:T9, "Test"=w188:dbl, "Warten"=w187:dbl)  [unwired: 5 in, 1 out]
            n108 = Not(x=w186) -> (.not. x?=w189:bool)
            n109 = case shown="True" w186 {
              frame False {
              }
              frame True {
                n110 = property on="Registerkarte" class="RKElem (strikt)"("Val(Sgnl)"=T2."Result" ("Registerkarte")) -> (error out=w193:errorcluster)  [unwired: 2 in, 1 out]
                n111 = call "FGV Interference.vi"("error in (no error)"=w193, "Aktion FGV Interference"=Aktion_FGV_Interference."Lesen") -> ("Tabelle"=w196:T1[][])  [unwired: 8 in, 5 out]
                n112 = local write "LIN Ausgabetabelle"(w196) -> ()
              }
            }
          }
        }
        "Testdauer" <- w153
        "Stabilisierungszeit" <- w152
        n113 = case shown="True" w146 {
          frame False {
          }
          frame True {
            n114 = property on="Gasliste vergleichen" class="Bool. (strikt)"("Val(Sgnl)"=TRUE) -> (error out=w164:errorcluster)  [unwired: 2 in, 1 out]
            n115 = call <vilib>:"Clear Errors.vi"("error in (no error)"=w164) -> ("error out"=w163:errorcluster)  [unwired: 5 in, 1 out]
            n116 = flat-sequence {
              tunnel: w163 -> [_]
              frame #0 {
              }
            }
          }
        }
        n117 = case shown="True" w143 {
          selector: w143 -> [_ w161]
          frame False {
          }
          frame True {
            n118 = property on="Systemeinstellung" class="Bool. (strikt)"("Val(Sgnl)"=w161) -> (error out=w162:errorcluster)  [unwired: 2 in, 1 out]
            n119 = call <vilib>:"Clear Errors.vi"("error in (no error)"=w162) -> ()  [unwired: 5 in, 2 out]
          }
        }
        n120 = Empty String/Path?(string/path=w159) -> (empty?=w160:bool)
        n121 = case shown="False" w160 {
          tunnel: w157 -> [w197 w200]
          tunnel: w159 -> [w199 _]
          tunnel: [w198 w200] -> w158
          frame False {
            n122 = call "Strings und Zeitstempel verknuepfen.vi"("String 1 hinzufügen"=w199, "Eingagns String"=w197) -> ("Verknüpfter String"=w198:string)  [unwired: 9 in]
          }
          frame True {
          }
        }
      }
      event "Gasliste vergleichen": Value Change {
        n123 = event-data() -> ()  [unwired: 1 in, 1 out]
        n124 = flat-sequence {
          tunnel: [w259] -> w227
          tunnel: w227 -> [w273]
          frame #0 {
            n125 = call "Index uebersetzen.vi"("Aktion"=Aktion_Index_uebersetzten."auswerten") -> ("Komponenten"=w256:T16)  [unwired: 9 in, 1 out]
            n126 = Unbundle By Name(w256) -> ("Komponente"=w253:T1, "Interferent 1"=w257:T1, "Interferent 2"=w258:T1, "Interferent 3"=w254:T1)
            n127 = local write "Komponente 1S:"(w253) -> ()
            n128 = local write "Interferent 1:"(w257) -> ()
            n129 = local write "Interferent 2:"(w258) -> ()
            n130 = local write "Interferent 3:"(w254) -> ()
          }
          frame #1 {
            n131 = control-ref of="Komponente:"() -> (w267:refnum<vi>)
            n132 = control-ref of="Komponente:"() -> (w268:refnum<vi>)
            n133 = control-ref of="Interferent 1:"() -> (w269:refnum<vi>)
            n134 = control-ref of="Interferent 2:"() -> (w260:refnum<vi>)
            n135 = control-ref of="Interferent 3:"() -> (w261:refnum<vi>)
            n136 = control-ref of="Komponente 1:"() -> (w270:refnum<vi>)
            n137 = control-ref of="Interferent 1: 2"() -> (w264:refnum<vi>)
            n138 = control-ref of="Interferent 2: 2"() -> (w263:refnum<vi>)
            n139 = control-ref of="Interferent 3: 2"() -> (w262:refnum<vi>)
            n140 = Build Array(w267) -> (w266:refnum<vi>[])
            n141 = Build Array(w268, w269, w260, w261) -> (w259:refnum<vi>[])
            n142 = Build Array(w270, w264, w263, w262) -> (w265:refnum<vi>[])
            n143 = call "dynEinheiten.vi"("Komponenten Ref."=w259, "Sollwert Ref."=w265) -> ()  [unwired: 10 in]
            n144 = call "dynEinheiten.vi"("Komponenten Ref."=w259, "Sollwert Ref."=w259) -> ()  [unwired: 10 in]
            n145 = call "dynEinheiten.vi"("Komponenten Ref."=w259, "Sollwert Ref."=w266) -> ()  [unwired: 10 in]
          }
          frame #2 {
            n146 = for {
              tunnel: w273 -> [w275] mode=indexing
              tunnel: [w274] -> w271 mode=indexing
              n147 = property class="Ring (strikt)"(reference=w275) -> ("Caption.Text"=w274:string)  [unwired: 1 in, 2 out]
            }
            n148 = call "FGV Interference.vi"("Êinheiten"=w271, "Aktion FGV Interference"=Aktion_FGV_Interference."Einheiten") -> ()  [unwired: 8 in, 6 out]
          }
        }
        n149 = Unbundle By Name("TestKonfig") -> ("Inter 1 aktiv"=w224:bool, "Inter 2 aktiv"=w205:bool, "Inter 3 aktiv"=w223:bool)
        n150 = control-ref of="Komponente 1:"() -> (w218:refnum<vi>)
        n151 = control-ref of="Interferent 1: 2"() -> (w219:refnum<vi>)
        n152 = control-ref of="Interferent 2: 2"() -> (w220:refnum<vi>)
        n153 = control-ref of="Interferent 3: 2"() -> (w221:refnum<vi>)
        n154 = control-ref of="Komponente 1S:"() -> (w217:refnum<vi>)
        n155 = control-ref of="Interferent 1:"() -> (w216:refnum<vi>)
        n156 = control-ref of="Interferent 2:"() -> (w215:refnum<vi>)
        n157 = control-ref of="Interferent 3:"() -> (w214:refnum<vi>)
        n158 = property on="Graph" class="SVDiagr (strikt)"("LegNumRows"=u32 4 ("Legende:Zeilenanzahl")) -> (error out=w226:errorcluster)  [unwired: 2 in, 1 out]
        n159 = Build Array(w218, w219, w220, w221) -> (w213:refnum<vi>[])
        n160 = Build Array(w217, w216, w215, w214) -> (w212:refnum<vi>[])
        n161 = Build Array(T11 TRUE ("Element"), w224, w205, w223) -> (w208:T11[])
        n162 = for {
          tunnel: w208 -> [w238] mode=indexing
          tunnel: w213 -> [w245] mode=indexing
          tunnel: w212 -> [w244] mode=indexing
          tunnel: [w243] -> w211 mode=indexing
          tunnel: [w242] -> w210 mode=indexing
          n163 = Select(t=T13."Enabled" ("Deaktiviert"), s=w238, f=T13."Disabled and Grayed Out" ("Deaktiviert")) -> (s? t:f=w239:T13)
          n164 = property class="DigWert (strikt)"(reference=w245, "DisabledEnum"=w239) -> (error out=w243:errorcluster)  [unwired: 1 in, 1 out]
          n165 = property class="Str (strikt)"(reference=w244, "DisabledEnum"=w239) -> (error out=w242:errorcluster)  [unwired: 1 in, 1 out]
        }
        n166 = for {
          shift-right: [w249] -> w222
          shift-left: w226 -> [w248]
          tunnel: w208 -> [w246] mode=indexing
          i -> [w247]
          n167 = property on="Graph" class="SVDiagr (strikt)"(error in=w248, "Active Plot"=w247) -> (error out=w250:errorcluster)  [unwired: 1 in, 1 out]
          n168 = property on="Graph" class="SVDiagr (strikt)"(error in=w250, "Plot.Visible?"=w246) -> (error out=w251:errorcluster)  [unwired: 1 in, 1 out]
          n169 = property on="Graph" class="SVDiagr (strikt)"(error in=w251, "ActYScl"=w247) -> (error out=w252:errorcluster)  [unwired: 1 in, 1 out]
          n170 = property on="Graph" class="SVDiagr (strikt)"(error in=w252, "YScale.Visible"=w246) -> (error out=w249:errorcluster)  [unwired: 1 in, 1 out]
        }
        n171 = case shown="True" w205 {
          tunnel: [w233 w236] -> _
          tunnel: [w230 w235] -> w203
          tunnel: "TestKonfig" -> [w232 w235]
          frame True {
            w231 = T6 0 items=["Messen", "CG zu PNS", "CG zu Entnahmestelle"] ("Wert")
            n172 = Bundle By Name(cluster=w232, "Komponente:"=w231) -> (w230:T5)
            n173 = property on="Modus" class="Ring (strikt)"("Value"=w231, "Disabled Items []"=i32[] [1, 2] ("Deaktivierte Objekte []")) -> (error out=w233:errorcluster)  [unwired: 2 in, 1 out]
          }
          frame False {
            n174 = property on="Modus" class="Ring (strikt)"("Disabled Items []"=i32[] [] ("Deaktivierte Objekte []")) -> (error out=w236:errorcluster)  [unwired: 2 in, 1 out]
          }
        }
        n175 = Merge Errors(w211, w210) -> (w209:errorcluster)
        n176 = call "Wertaenderung Gasliste.vi"("Aktion"=Aktion_Wertaenderung_Gasliste."Interference 375 inaktiv") -> ()  [unwired: 13 in, 2 out]
        n177 = call <vilib>:"Clear Errors.vi"("error in (no error)"=w222) -> ()  [unwired: 5 in, 2 out]
        n178 = call "FGV Interference.vi"("TestKonfig"=w203, "Aktion FGV Interference"=Aktion_FGV_Interference."TestKonfig") -> ()  [unwired: 8 in, 6 out]
        n179 = call <vilib>:"Clear Errors.vi"("error in (no error)"=w209) -> ()  [unwired: 5 in, 2 out]
      }
      event Value Change {
        n180 = event-data() -> ()  [unwired: 1 in, 1 out]
        n181 = call "FGV Interference.vi"("TestSetting"="TestSetting", "Aktion FGV Interference"=Aktion_FGV_Interference."TestSetting") -> ()  [unwired: 8 in, 6 out]
      }
      event "Test Start": Value Change {
        n182 = event-data() -> ()  [unwired: 1 in, 6 out]
        n183 = call "Test Status.vi"("Aktion"=Aktion_Test_Status."lesen") -> ("Tests sperren"=w282:bool)  [unwired: 11 in, 3 out]
        n184 = case shown="True" w282 {
          tunnel: [TRUE FALSE] -> w285
          tunnel: w281 -> [_ w287]
          frame False {
          }
          frame True {
            n185 = call "Texte in VIs uebersetzen.vi"("Sprachliste"=w287, "String zum Übersetzen"="Anderer Test läuft gerade.\nBitte etwas Geduld." ("Nachricht")) -> ("String zum Übersetzen"=w290:string)  [unwired: 9 in, 4 out]
            n186 = One Button Dialog(message=w290, button name ("OK")="OK" ("Schaltflächentext (\"OK\")")) -> ()  [unwired: 1 out]
          }
        }
      }
      event "Abbrechen": Value Change {
        n187 = event-data() -> ()  [unwired: 1 in, 3 out]
        n188 = call "Test Status.vi"("Aktion"=Aktion_Test_Status."lesen") -> ("Aktive Tests"=w296:T24, "Tests sperren"=w294:bool)  [unwired: 11 in, 2 out]
        n189 = Unbundle By Name(w296) -> ("Interference 375 läuft"=w295:bool)
        n190 = And(x=w295, y=w294) -> (x .and. y?=w293:bool)
        n191 = case shown="True" w293 {
          tunnel: [w304 w313] -> w302
          tunnel: w301 -> [w304 w312]
          tunnel: [w303 FALSE] -> w299
          tunnel: w298 -> [_ w305]
          tunnel: w292 -> [w303 _]
          frame False {
          }
          frame True {
            n192 = call "FGV-Funktionstasten.vi"("Herkunft"="Interference Test", "Zustand"=Zustaende."Standby", "Aktion"=Funktionstasten-Aktion."Zustand setzen") -> ()  [unwired: 5 in, 8 out]
            n193 = call "Texte in VIs uebersetzen.vi"("Sprachliste"=w305, "String zum Übersetzen"="Test abgebrochen" ("String 1 hinzufügen")) -> ("String zum Übersetzen"=w306:string)  [unwired: 9 in, 4 out]
            n194 = call "Strings und Zeitstempel verknuepfen.vi"("String 1 hinzufügen"=w306, "Eingagns String"=w312) -> ("Verknüpfter String"=w313:string)  [unwired: 9 in]
          }
        }
      }
      event "Daten löschen": Value Change {
        n195 = event-data() -> ()  [unwired: 1 in, 3 out]
        n196 = flat-sequence {
          frame #0 {
            n197 = call "FGV Interference.vi"("Aktion FGV Interference"=Aktion_FGV_Interference."löschen") -> ("Tabelle"=w317:T1[][])  [unwired: 9 in, 5 out]
            n198 = local write "LIN Ausgabetabelle"(w317) -> ()
          }
          frame #1 {
            n199 = call "Auswerten.vi"() -> ("Konzentration Komponente"=w318:dbl, "Komponente:"=w320:T1, "max. Flow Weighted Mean:"=w321:T1, "Konzentration FlowWeightedMean"=w319:dbl)  [unwired: 8 in]
            n200 = local write "[ppm]"(w318) -> ()
            n201 = local write "Konzentration FlowWeightedMean"(w319) -> ()
            n202 = local write "max. Flow Weighted Mean:"(w321) -> ()
            n203 = local write "Komponente:"(w320) -> ()
            n204 = local write "Konzentration Komponente"(w318) -> ()
          }
          frame #2 {
            n205 = control-ref of="LIN Ausgabetabelle"() -> (w323:refnum<vi>)
            n206 = call "Zeile faerben.vi"("Anzahl"=5, "Table (Eingang)"=w323) -> ()  [unwired: 9 in, 1 out]
          }
        }
      }
      event "Print to PDF": Value Change {
        n207 = event-data() -> ()  [unwired: 1 in, 1 out]
        n208 = call "FGV Interference.vi"("Aktion FGV Interference"=Aktion_FGV_Interference."Lesen") -> ("TestSetting"=w334:T3)  [unwired: 9 in, 5 out]
        n209 = Unbundle By Name(w334) -> ("Pfad:"=w333:path, "Textname:"=w332:string)
        n210 = Concatenate Strings(w332, ".pdf") -> (w340:string)
        n211 = Build Path(base path=w333, name or relative path=w340) -> (appended path=w324:path)
        n212 = disable-structure shown="BullZip==TRUE" {
          disable-tunnel: w324 -> [w349 _]
          disable-tunnel: [w348 _] -> w331
          frame condition #0 {
            n213 = call "Save to PDF File using BullZip 2009.vi"("Save PDF File Path"=w349) -> ("error out"=w348:errorcluster)  [unwired: 10 in]
          }
          frame condition #1 (active) {
          }
        }
        n214 = disable-structure shown="Aktiviert" {
          disable-tunnel: w331 -> [w342 w345]
          disable-tunnel: [w341 w344] -> w325
          disable-tunnel: w324 -> [_ w343]
          frame Disabled {
            n215 = call "PDF Protokoll EPA1065_InterferenceVerification.vi"("error in (no error)"=w342) -> ("error out"=w341:errorcluster)  [unwired: 10 in]
          }
          frame Enabled {
            # "#PDF_Interface"
            n216 = call "PDF_Interface_PDF Protokoll EPA1065_InterferenceVerification.vi"("error in (no error)"=w345, "Save PDF File Path"=w343) -> ("error out"=w344:errorcluster)  [unwired: 9 in]
          }
        }
        n217 = case shown="Fehler" w325 {
          tunnel: ["Daten gespeichert!" ("String") "Fehler beim schreiben der Daten" ("String")] -> w329
          frame No Error {
          }
          frame Error {
          }
        }
        n218 = call <vilib>:"Clear Errors.vi"("error in (no error)"=w325) -> ()  [unwired: 5 in, 2 out]
        n219 = call "Tabelle in die einzelnen Seiten zerlegen.vi"("Aktion"=FGV_Aktion_Tabelle_zerlegen."vereinzeln", "Index (Seite)"=38) -> ("Sprachliste"=w328:string[][])  [unwired: 7 in, 2 out]
        n220 = call "Texte in VIs uebersetzen.vi"("Sprachliste"=w328, "String zum Übersetzen"=w329) -> ("String zum Übersetzen"=w330:string)  [unwired: 9 in, 4 out]
        n221 = One Button Dialog(message=w330) -> ()  [unwired: 1 in, 1 out]
      }
      event "Systemeinstellung": Value Change {
        n222 = event-data() -> ()  [unwired: 1 in, 1 out]
        n223 = stacked-sequence {
          frame #0 {
          }
          frame #1 {
            n224 = control-ref of="Analysator"() -> (w353:refnum<vi>)
            n225 = call "Analysator initialisieren.vi"("Referenz Analysator"=w353) -> ()  [unwired: 9 in, 2 out]
          }
          frame #2 {
            n226 = call "Wertaenderung Systemeinstellungen.vi"("Aktion"=Aktion_Wertaenderung_Gasliste."Interference 375 inaktiv") -> ()  [unwired: 13 in, 2 out]
            n227 = local write "Systemeinstellung"(FALSE ("Systemeinstellung")) -> ()
          }
        }
      }
      event "Save to file": Value Change {
        n228 = event-data() -> ()  [unwired: 1 in, 1 out]
        n229 = call "FGV Interference.vi"("Aktion FGV Interference"=Aktion_FGV_Interference."Lesen") -> ("TestSetting"=w374:T3)  [unwired: 9 in, 5 out]
        n230 = Unbundle By Name(w374) -> ("Pfad:"=w373:path, "Textname:"=w372:string)
        n231 = Concatenate Strings(w372, ".txt") -> (w377:string)
        n232 = Build Path(base path=w373, name or relative path=w377) -> (appended path=w361:path)
        n233 = Open/Create/Replace File(file path (use dialog)=w361, operation (0:open)=T22."replace or create with confirmation" ("Operation (0:Öffnen)")) -> (refnum out=w363:refnum<file>, error out=w364:errorcluster)  [unwired: 4 in, 1 out]
        n234 = call "Interference 1065.375 Textfile.vi"() -> ("Textfile"=w359:string[])  [unwired: 11 in]
        n235 = Write to Text File(file (use dialog)=w363, text=w359, error in=w364) -> (refnum out=w366:refnum<file>, error out=w360:errorcluster)  [unwired: 1 in, 1 out]
        n236 = case shown="Fehler" w360 {
          tunnel: ["Daten gespeichert!" ("String") "Fehler beim schreiben der Daten" ("String")] -> w370
          frame No Error {
          }
          frame Error {
          }
        }
        n237 = Close File(refnum=w366, error in=w360) -> (error out=w365:errorcluster)  [unwired: 1 out]
        n238 = call <vilib>:"Clear Errors.vi"("error in (no error)"=w365) -> ()  [unwired: 5 in, 2 out]
        n239 = call "Tabelle in die einzelnen Seiten zerlegen.vi"("Aktion"=FGV_Aktion_Tabelle_zerlegen."vereinzeln", "Index (Seite)"=38) -> ("Sprachliste"=w369:string[][])  [unwired: 7 in, 2 out]
        n240 = call "Texte in VIs uebersetzen.vi"("Sprachliste"=w369, "String zum Übersetzen"=w370) -> ("String zum Übersetzen"=w371:string)  [unwired: 9 in, 4 out]
        n241 = One Button Dialog(message=w371) -> ()  [unwired: 1 in, 1 out]
      }
      event "Speichern", "Speichern 2": Value Change {
        n242 = event-data() -> ()  [unwired: 1 in, 6 out]
        n243 = call "FGV Interference.vi"("Aktion FGV Interference"=Aktion_FGV_Interference."Speichern") -> ()  [unwired: 9 in, 6 out]
      }
      event "Graph löschen": Value Change {
        n244 = event-data() -> ()  [unwired: 1 in, 3 out]
        n245 = property on="Graph" class="SVDiagr (strikt)"("History Data"=waveform(dbl)[][] [] ("Historiendaten")) -> (error out=w388:errorcluster)  [unwired: 2 in, 1 out]
        n246 = call <vilib>:"Clear Errors.vi"("error in (no error)"=w388) -> ()  [unwired: 5 in, 2 out]
        n247 = call "FGV Messdaten.vi"("Aktionen"=Aktionen_FGV_Messdaten."löschen") -> ()  [unwired: 6 in, 9 out]
      }
      event "Registerkarte": Value Change {
        n248 = event-data() -> ()  [unwired: 1 in, 6 out]
        n249 = flat-sequence {
          tunnel: [w418] -> w407
          tunnel: [w413] -> w394
          frame #0 {
            n250 = control-ref of="LIN Ausgabetabelle"() -> (w409:refnum<vi>)
            n251 = call "Zeile faerben.vi"("Anzahl"=5, "Table (Eingang)"=w409) -> ()  [unwired: 9 in, 1 out]
          }
          frame #1 {
            n252 = control-ref of="LIN Ausgabetabelle"() -> (w422:refnum<vi>)
            n253 = control-ref of="max. Flow Weighted Mean:"() -> (w424:refnum<vi>)
            n254 = control-ref of="Komponente:"() -> (w423:refnum<vi>)
            n255 = call "FGV Interference.vi"("Aktion FGV Interference"=Aktion_FGV_Interference."Lesen") -> ("Êinheiten"=w421:string[], "Tabelle"=w418:T1[][])  [unwired: 9 in, 4 out]
            n256 = call "Auswerten.vi"("Êinheiten"=w421, "LIN Ausgabetabelle"=w422, "Komponente:"=w423, "max. Flow Weighted Mean:"=w424, "Tabelle"=w418) -> ("Konzentration Komponente"=w410:dbl, "Komponente:"=→"Komponente:":T1, "max. Flow Weighted Mean:"=→"max. Flow Weighted Mean:":T1, "Konzentration FlowWeightedMean"=→"Konzentration FlowWeightedMean":dbl)  [unwired: 3 in]
            "Konzentration Komponente" <- w410
            "[ppm]" <- w410
            n257 = disable-structure shown="Aktiviert" {
              disable-tunnel: [w427 w428] -> w417
              disable-tunnel: w410 -> [w426 w428]
              frame Disabled {
                n258 = Absolute Value(x=w426) -> (abs(x)=w427:dbl)
              }
              frame Enabled {
              }
            }
            n259 = Less Or Equal?(x=w417, y=1.0) -> (x <= y?=w415:bool)
            n260 = Not A Number/Path/Refnum?(number/path/refnum=w417) -> (NaN/Path/Refnum?=w416:bool)
            n261 = Not(x=w416) -> (.not. x?=w414:bool)
            n262 = And(x=w414, y=w415) -> (x .and. y?=w413:bool)
          }
        }
        n263 = property on="Tabelle 3" class="Tbl (strikt)"("Active Cell"=T23 {"Row"=0, "Column"=1} ("Aktive Zelle:Aktive Zelle")) -> (error out=w400:errorcluster)  [unwired: 2 in, 1 out]
        n264 = Select(t=u32 6618880, s=w394, f=u32 16711680) -> (s? t:f=w401:u32)
        n265 = property on="Tabelle 3" class="Tbl (strikt)"(error in=w400, "Cell BG Color"=w401) -> (error out=w395:errorcluster)  [unwired: 1 in, 1 out]
        n266 = property on="Tabelle 3" class="Tbl (strikt)"(error in=w395, "Active Cell"=T23 {"Row"=0, "Column"=1} ("Aktive Zelle:Aktive Zelle")) -> ()  [unwired: 1 in, 2 out]
        n267 = Select(t=string[][] [["EPA §1065.375 Interference verification of N2O"], ["Passed"]] ("Tabelle 3"), s=w394, f=string[][] [["EPA §1065.375 Interference verification of N2O"], ["NOT Passed"]] ("Tabelle 3")) -> (s? t:f=w391:string[][])
        n268 = call "Texte in VIs uebersetzen.vi"("Sprachliste"=w392, "2D String-Array zum Übersetzen"=w391) -> ("2D String-Array zum Übersetzen"=w393:string[][])  [unwired: 9 in, 4 out]
        n269 = Transpose 2D Array(2D array=w393) -> (transposed array=→"Tabelle 3":string[][])
        "LIN Ausgabetabelle" <- w407
      }
    }
    "Status" <- w135
    n270 = Not Equal?(x=w137, y=w135) -> (x != y?=w136:bool)
    n271 = case shown="False" w136 {
      frame False {
      }
      frame True {
        n272 = property on="Status" class="Str"("Text.Scroll Position"=u32 9999 ("Text.Anzeigeposition")) -> (error out=w430:errorcluster)  [unwired: 2 in, 1 out]
        n273 = call <vilib>:"Clear Errors.vi"("error in (no error)"=w430) -> ()  [unwired: 5 in, 2 out]
      }
    }
  }
